vi "get_cluster_element_regions.vi"(9 "cluster offset":i32, 11 "TypeDescriptor":refnum<class "TD.lvclass">) -> (1 "offset past element TDs":i32, 2 "element_regions":cluster{i32, i32}[](array[cluster]), 3 "TypeDescriptor out":refnum<class "TD.lvclass">)   [LabVIEW 2020, in "variant.lvlib" / "type.lvlib" / "TD.lvclass"]
uses:
  TD.lvclass
  C:/projects/OpenG-Variant-Data-Library/source/library/Bytes/Bytes.lvclass
  Bytes/Bytes.lvclass/Bytes.ctl
  88692a85-5cdd-45bb-8e9c-48d4fd1ea210.vi
  get_num_elements.vi/b3898c1b-5169-4cb1-894b-457c92b4a1c3.vi
  88692a85-5cdd-45bb-8e9c-48d4fd1ea210.vi/81433c74-ee36-47cf-a886-10c868675b30.vi
  88692a85-5cdd-45bb-8e9c-48d4fd1ea210.vi/d8d9ff34-2c15-4edb-a5ad-7260f11560db.vi
  Bytes/read.vi
  get_num_elements.vi/b3898c1b-5169-4cb1-894b-457c92b4a1c3.vi/81433c74-ee36-47cf-a886-10c868675b30.vi
  get_num_elements.vi/b3898c1b-5169-4cb1-894b-457c92b4a1c3.vi/d8d9ff34-2c15-4edb-a5ad-7260f11560db.vi
  Bytes/to_data.vi
  Bytes/from_byte_array.vi
  Bytes/Bytes.lvclass
  TD.lvclass/TD.ctl
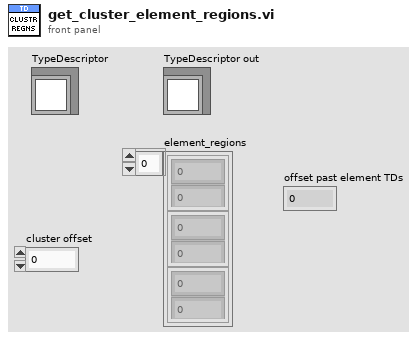
[diagram p1: front panel]
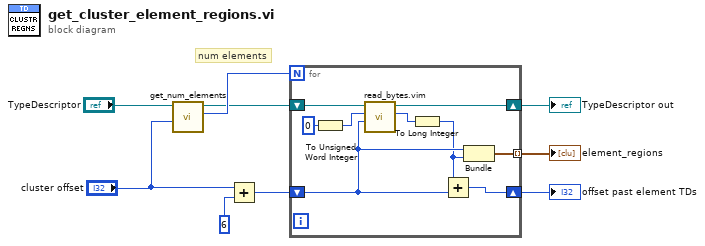
[diagram p0: block diagram]
diagram:
  # "num elements"
  n1 = call "get_num_elements.vi"("item offset"="cluster offset", "TypeDescriptor"="TypeDescriptor") -> ("num_element"=w7:i32, "TypeDescriptor out"=w6:refnum<class "TD.lvclass">)  [unwired: 8 in]
  n2 = Add(x="cluster offset", y=6) -> (x+y=w2:i32)
  n3 = for {
    N: w7 -> [_]
    shift-right: [w15] -> w5
    shift-left: w2 -> [w12]
    shift-right: [w14] -> w9
    shift-left: w6 -> [w18]
    tunnel: [w10] -> w4 mode=indexing
    n4 = To Unsigned Word Integer(number=u8 0) -> (unsigned 16bit integer=w16:u16)
    n5 = call "read_bytes.vim"("byte offset"=w12, "data type"=w16, "Bytes in"=w18) -> ("value"=w13:u16, "Bytes out"=w14:refnum<class "TD.lvclass">)  [unwired: 7 in]
    n6 = To Long Integer(number=w13) -> (32bit integer=w11:i32)
    n7 = Add(x=w11, y=w12) -> (x+y=w15:i32)
    n8 = Bundle(w12, w11) -> (w10:cluster{i32, i32})  [unwired: 1 in]
  }
  "TypeDescriptor out" <- w9
  "offset past element TDs" <- w5
  "element_regions" <- w4
